vi "InitWaveform.vi"() -> (3 "output waveform":waveform(dbl))   [LabVIEW 2016]
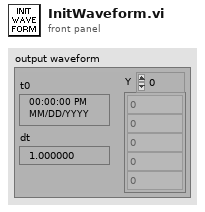
[diagram p1: front panel]
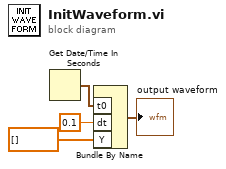
[diagram p0: block diagram]
diagram:
  n1 = Get Date/Time In Seconds() -> (seconds since 1Jan1904=w2:timestamp)
  n2 = Bundle By Name("t0"=w2, "dt"=0.1, "Y"=dbl[] []) -> (→"output waveform":waveform(dbl))  [unwired: 1 in]
